vi "getSpeed.vi"(3 "ID":i32, 4 "handle":i32, 5 "错误输入（无错误）":errorcluster) -> (0 "return":sgl, 1 "错误输出":errorcluster)   [LabVIEW 2013, in "EM_CVx.lvlib"]
uses:
  EM_CVx.lvlib
  library/moverLibrary_x86.dll
  library/moverLibrary_x64.dll
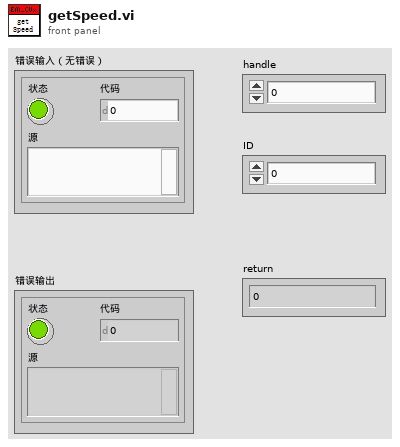
[diagram p1: front panel]
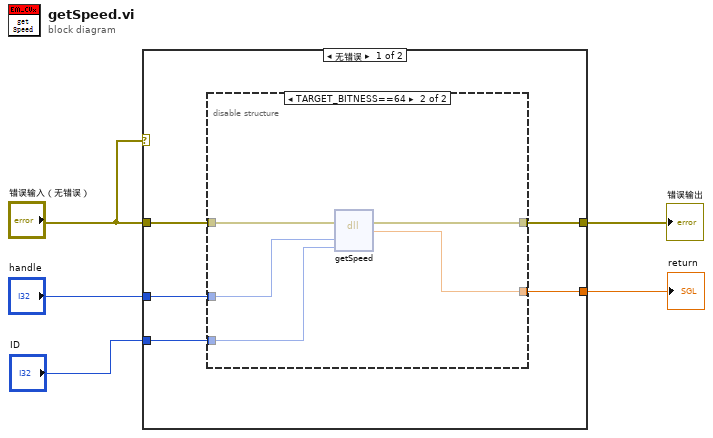
[diagram p0: block diagram]
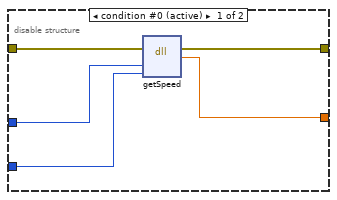
[diagram p2: hidden frame]
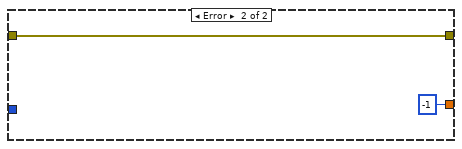
[diagram p3: hidden frame]
diagram:
  n1 = case shown="无错误" "错误输入（无错误）" {
    tunnel: "错误输入（无错误）" -> [w10 w22]
    tunnel: "handle" -> [w9 _]
    tunnel: "ID" -> [w8 _]
    tunnel: [w7 w22] -> w3
    tunnel: [w6 -1 ("state")] -> w2
    frame No Error {
      n2 = disable-structure shown="TARGET_BITNESS==64" {
        disable-tunnel: w10 -> [w15 w20]
        disable-tunnel: w9 -> [w14 w18]
        disable-tunnel: w8 -> [w13 w17]
        disable-tunnel: [w12 w19] -> w7
        disable-tunnel: [w11 w16] -> w6
        frame condition #0 (active) {
          n3 = dll-call lib="E:/5-mover/4-labView/EM_CVx_2013/library/moverLibrary_x86.dll" fn="getSpeed"(error in=w15, "handle"=w14, "ID"=w13) -> (error out=w12:errorcluster, "return"=w11:sgl)  [unwired: 4 in, 1 out]
        }
        frame condition #1 {
          n4 = dll-call lib="E:/5-mover/4-labView/EM_CVx_2013/library/moverLibrary_x64.dll" fn="getSpeed"(error in=w20, "handle"=w18, "ID"=w17) -> (error out=w19:errorcluster, "return"=w16:sgl)  [unwired: 4 in, 1 out]
        }
      }
    }
    frame Error {
    }
  }
  "错误输出" <- w3
  "return" <- w2
